vi "Close.vi"(8 "error in (no error)":errorcluster, 11 "Osciloscope in":refnum<class "Osciloscope.lvclass">) -> (0 "error out":errorcluster, 3 "Osciloscope out":refnum<class "Osciloscope.lvclass">)   [LabVIEW 2020, in "Controlador.lvlib" / "Osciloscope.lvclass"]
uses:
  Osciloscope.lvclass
  Osciloscope.lvclass/Osciloscope.ctl
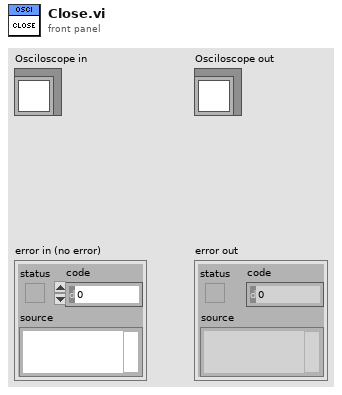
[diagram p1: front panel]
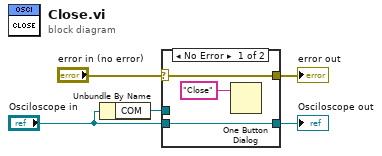
[diagram p0: block diagram]
diagram:
  n1 = Unbundle By Name("Osciloscope in") -> ("COM"=w1:refnum<visa-resource-name>)
  n2 = case shown="No Error" "error in (no error)" {
    selector: "error in (no error)" -> [w7 w10]
    tunnel: [w7 w10] -> w4
    tunnel: [w8 w9] -> w3
    tunnel: "Osciloscope in" -> [w8 w9]
    tunnel: w1 -> [_ _]
    frame No Error {
      n3 = One Button Dialog(message="Close") -> ()  [unwired: 1 in, 1 out]
    }
    frame Error {
    }
  }
  "error out" <- w4
  "Osciloscope out" <- w3
